vi "Test 6.vi"() -> ()   [LabVIEW 2015, in "Drona basic.lvlib"]
uses:
  Drona basic.lvlib
  <vilib>/Utility/miscctls.llb/LVPoint32TypeDef.ctl
  <vilib>/Utility/miscctls.llb/LVPositionTypeDef.ctl
  <vilib>/Utility/miscctls.llb/LVBoundsTypeDef.ctl
panel:
  in  "Tab Control 2":enum32{"Page 1", "Page 2"}(tab)
  in  "Tab Control":enum32{"Page 1", "Page 2"}(tab)
  in  "Boolean":bool
  out "Button":u16
  out "Coords":T1
  out "Position":T2
  out "Bounds":T3
  in  "Numeric":dbl
  in  "Cluster":T4
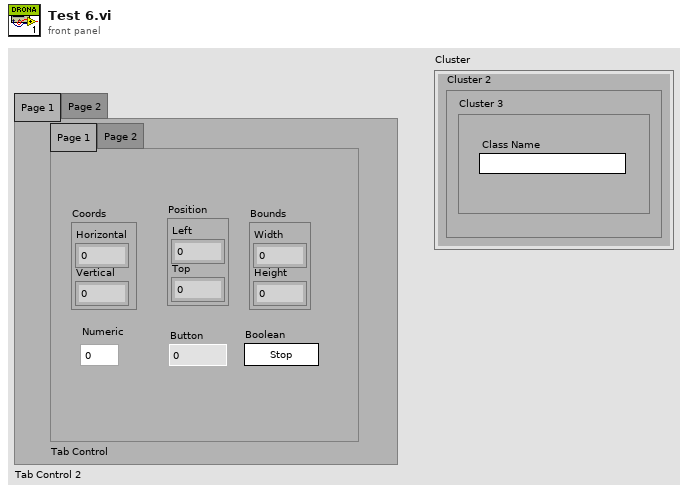
[diagram p1: front panel]
types:
  T1 = typedef "LVPoint32TypeDef.ctl" = cluster{"Horizontal":i32, "Vertical":i32}
  T2 = typedef "LVPositionTypeDef.ctl" = cluster{"Left":i32, "Top":i32}
  T3 = typedef "LVBoundsTypeDef.ctl" = cluster{"Width":u32, "Height":u32}
  T4 = cluster{"Cluster 2":cluster{"Cluster 3":cluster{"Class Name":string}}}
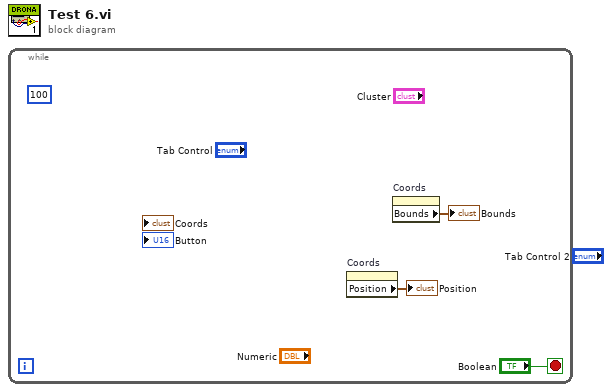
[diagram p0: block diagram]
diagram:
  n1 = while {
    stop <- "Boolean" stop-if-true
    (unwired) 100
    n2 = property on="Coords" class="Clust (strict)"() -> ("Position"=→"Position":T2)  [unwired: 2 in, 2 out]
    n3 = property on="Coords" class="Clust (strict)"() -> ("Bounds"=→"Bounds":T3)  [unwired: 2 in, 2 out]
  }
